vi "Write Error to Log.vi"(8 "error in (no error)":errorcluster, 11 "file reference in":refnum<file>) -> (0 "error out":errorcluster, 3 "file reference out":refnum<file>)   [LabVIEW 2024]
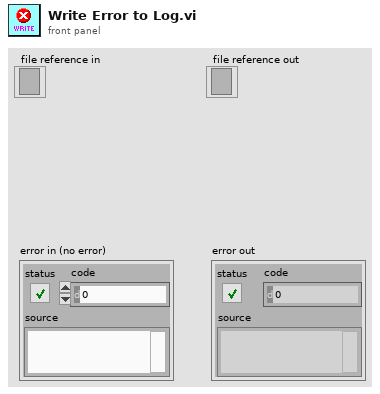
[diagram p1: front panel]
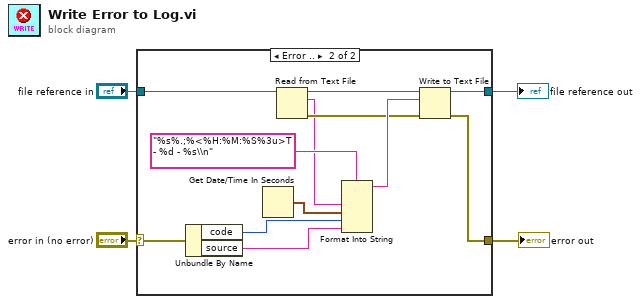
[diagram p0: block diagram]
diagram:
  n1 = case shown="Error .." "error in (no error)" {
    selector: "error in (no error)" -> [w6 w13]
    tunnel: "file reference in" -> [w5 w10]
    tunnel: [w5 w18] -> w3
    tunnel: [w6 w17] -> w2
    frame No Error {
    }
    frame Error {
      n2 = Unbundle By Name(w13) -> ("code"=w12:i32, "source"=w11:string)
      n3 = Get Date/Time In Seconds() -> (seconds since 1Jan1904=w15:timestamp)
      n4 = Read from Text File(file (use dialog)=w10) -> (refnum out=w9:refnum<file>, text=w7:string, error out=w8:errorcluster)  [unwired: 3 in, 1 out]
      n5 = Format Into String(format string="%s%.;%<%H:%M:%S%3u>T - %d - %s\\n" ("Local Time"), w7, w15, w12, w11) -> (resulting string=w14:string)  [unwired: 2 in, 1 out]
      n6 = Write to Text File(file (use dialog)=w9, text=w14, error in=w8) -> (refnum out=w18:refnum<file>, error out=w17:errorcluster)  [unwired: 1 in, 1 out]
    }
  }
  "file reference out" <- w3
  "error out" <- w2
